vi "Teleop.vi"(10 "Match Info":T1={"Autonomous Elapsed Seconds"=0.0, "TeleOp Elapsed Seconds"=0.0, "Disabled Elapsed Seconds"=0.0, "Visited Autonomous"=FALSE, "Visited TeleOp"=FALSE, "Visited Disabled"=FALSE, "Autonomous Settings"={"Autonomous Style"=enum."Independent", "VI Refnum"=refnum}}, 11 "Call Context":T2) -> ()   [LabVIEW 2014]
doc: "This VI is called for each TeleOp packet received from the DS where the robot is not disabled. It is often used to read from the joysticks and update I/O or to update setpoints for timed control loops. It should complete and return within 20 milliseconds or it may miss DS packets."
uses:
  <vilib>/Rock Robotics/WPI/DriverStation/WPI_DriverStationDerivedRobotMode.ctl
  <vilib>/Rock Robotics/WPI/DriverStation/WPI_DriverStationMatch Info.ctl
  Drivetrain Code/Drivetrain Control.ctl
  Drivetrain Code/Drivetrain Mode.ctl
  Common Code/Change Detect.vi
  Common Code/Change Detect Boolean.vi
  <vilib>/Rock Robotics/WPI/Joystick/WPI_JoystickGetSetRefNum.vi
  Robot Global Data.vi
  <vilib>/Rock Robotics/WPI/Solenoid/Deprecated/WPI_SolenoidSetBool.vi
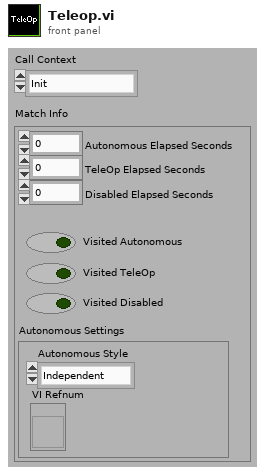
[diagram p1: front panel]
types:
  T1 = typedef "WPI_DriverStationMatch Info.ctl" = cluster{"Autonomous Elapsed Seconds":dbl, "TeleOp Elapsed Seconds":dbl, "Disabled Elapsed Seconds":dbl, "Visited Autonomous":bool, "Visited TeleOp":bool, "Visited Disabled":bool, "Autonomous Settings":cluster{"Autonomous Style":enum16{"Iterative", "Independent"}, "VI Refnum":refnum<vi>}}
  T2 = typedef "WPI_DriverStationDerivedRobotMode.ctl" = enum16{"Init", "Execute", "Stop"}
  T3 = enum16{"0", "1", "2", "3", "4", "5", "6", "7", "8", "9", "A", "B", "C", "D", "E", "F", "G", "H", "I", "J", "K", "L", "M", "N", "O", "P", "Q", "R", "S", "T", "U", "V", "W", "X", "Y", "Z", "F1", "F2", "F3", "F4", "F5", "F6", "F7", "F8", "F9", "F10", "F11", "F12", "F13", "F14", "F15", "ADD", "BACK", "BACKSLASH", "CAPITAL", "COMMA", "DECIMAL", "DELETE", "DIVIDE", "DOWN", "END", "EQUALS", "ESCAPE", "GRAVE (`)", "HOME", "INSERT", "LBRACKET", "LCONTROL", "LEFT", "L ALT", "LSHIFT", "LWIN", "MINUS", "MULTIPLY", "NEXT", "NUMLOCK", "NUMPAD_0", "NUMPAD_1", "NUMPAD_2", "NUMPAD_3", "NUMPAD_4", "NUMPAD_5", "NUMPAD_6", "NUMPAD_7", "NUMPAD_8", "NUMPAD_9", "PAUSE", "PERIOD", "PRIOR (PG UP)", "RBRACKET", "RCONTROL", "RETURN", "RIGHT", "R ALT", "RSHIFT", "RWIN", "SCROLL", "SEMICOLON", "SLASH", "SPACE", "SUBTRACT", "TAB", "UP", "ENTER (num pad)", "' (quote)"}
  T4 = typedef "Drivetrain Mode.ctl" = enum16{"Manual", "Gyro Steer", "Vision Steer", "Drive Distance", "Yaw Rate Compensate"}
  T5 = typedef "Drivetrain Control.ctl" = cluster{"Mode":T4, "Steer":dbl, "Y":dbl, "Heading Target":dbl, "Strafe X":dbl, "Y Target":dbl, "Strafe Target":dbl, "X Max Speed":dbl, "X Min Speed":dbl, "Y Max Speed":dbl, "Y Min Speed":dbl, "Force strafe":bool, "Pivot Speed":dbl}
  T6 = typedef "WPI_JoystickDevRef.ctl" = cluster{"Device":T7}
  T7 = typedef "WPI_JoystickDeviceEnum.ctl" = enum16{"USB 0", "USB 1", "USB 2", "USB 3", "USB 4", "USB 5"}
  T8 = typedef "D-Pad.ctl" = cluster{"Top":bool, "Bottom":bool, "None":bool, "Right":bool, "Left":bool}
  T9 = typedef "Button Cluster.ctl" = cluster{"Buttons[0]":bool, "Buttons[1]":bool, "Buttons[2]":bool, "Buttons[3]":bool, "Buttons[4]":bool, "Buttons[5]":bool, "Buttons[6]":bool, "Buttons[7]":bool, "Buttons[8]":bool, "Buttons[9]":bool}
  T10 = typedef "Axes Cluster.ctl" = cluster{"Axes[0]":dbl, "Axes[1]":dbl, "Axes[2]":dbl, "Axes[3]":dbl, "Axes[4]":dbl, "Axes[5]":dbl, "Axes[6]":dbl, "Axes[7]":dbl, "Axes[8]":dbl}
  T11 = typedef "Dashboard Control Data.ctl" = cluster{"Cam Exposure":dbl, "Go to angle":dbl, "Steer PID Gains":cluster{"proportional gain (Kc)":dbl, "integral time (Ti, min)":dbl, "derivative time (Td, min)":dbl}, "Steer PID output Range":cluster{"output high":dbl, "output low":dbl}, "Pressure m \nValue":dbl, "Pressure b \nValue":dbl, "Roller Command Cluster ":T12, "Elevator":T13, "Encoder Control":T15, "Auton Settings":cluster{"Drive Dist Window Size":dbl}, "Drivetrain Settings":T16, "Lance":T17}
  T12 = typedef "Roller Control.ctl" = cluster{"Intake Speed":dbl, "Turn In Speed":dbl, "Unload Speed":dbl, "Turn Out Speed":dbl, "Ping Align Tolerance":dbl, "Tote Range Threshold":dbl, "Right Pot 0":dbl, "Pot Threshold":dbl, "Left Pot 0":dbl, "Right Pot Scale":dbl, "Left Pot Scale":dbl, "Min Elevator Height":dbl, "Eject Time":dbl, "Eject US Threshold":dbl, "Anti-Twitch Time":u32, "Ping Caring Threshold":dbl, "Pot Diff Threshold":dbl, "Pinch Sustain":u32, "Absorb Give Up Threshold":dbl, "Untip In Threshold":dbl, "Untip Grab Range":dbl, "Ultrasonic Hold Time":u32, "Landscape Absorb Time":u32, "Pot Use Wait Time":u32, "Can Turn Stop Range":dbl, "HP Load Speed":dbl, "Stick Multiplier":dbl, "Coop Eject Speed":dbl}
  T13 = typedef "Elevator DB Control.ctl" = cluster{"PID Output Range":cluster{"output high":dbl, "output low":dbl}, "PID gains":cluster{"proportional gain (Kc)":dbl, "integral time (Ti, min)":dbl, "derivative time (Td, min)":dbl}, "Height Tolerance":sgl, " Encoder Constant":dbl, "Eject Time":sgl, "Zeroing Speed":sgl, "Presets":T14, "Ping Detect Threshold":sgl, "Trashcan Detect Threshold":sgl, "Zero Filter Time":dbl, "Stabilizer Open Time":dbl, "Zero Creep Speed":dbl, "Max Current":dbl, "Current Trip Time":dbl, "Abort Pitch":dbl, "Finger m":dbl, "Finger b":dbl, "Finger max ":dbl, "Finger Stabilizer":dbl, "Finger Store":dbl, "Finger Stop Store":dbl, "Stabilizer Close Time":dbl, "Finger min":dbl, "Unstick gain":dbl, "Full Detect Max":dbl}
  T14 = typedef "Elevator Presets.ctl" = cluster{"Pickup 2 w/ Tote":sgl, "Pickup 2 w/ Trashcan":sgl, "Pickup 3 w/ Tote":sgl, "Pickup 3 w/ Trashcan":sgl, "Bottom":sgl, "Pickup 1 w/ Tote":sgl, "Pickup Trashcan":sgl, "Pickup 1 w/ Trashcan":sgl, "Eject":sgl, "Hold Low":sgl, "Step add height":sgl, "Untip Lift":dbl, "Drop Stack":dbl, "HP Load Hold":dbl, "HP Load Drop":dbl, "HP Load Hold Can":dbl, "Store can max":dbl, "HP Drag Score":dbl, "HP Drag Finish":dbl, "Finger trashcan avoid":dbl, "Full":dbl}
  T15 = typedef "Encoder Control.ctl" = cluster{"Left Tick Constant":dbl, "Right Tick Constant":dbl, "Center Tick Constant":dbl, "Reset?":bool, "Y Dist":cluster{"PID gains":cluster{"proportional gain (Kc)":dbl, "integral time (Ti, min)":dbl, "derivative time (Td, min)":dbl}}, "X Dist":cluster{"PID gains":cluster{"proportional gain (Kc)":dbl, "integral time (Ti, min)":dbl, "derivative time (Td, min)":dbl}}, "Y Stop Thresh":dbl, "Y Stop Speed":dbl, "X Stop Thresh":dbl, "X Stop Speed":dbl}
  T16 = typedef "Drivetrain Settings.ctl" = cluster{"Gyro Tolerance":sgl, "Strafe Correct max steer":sgl, "Strafe Timer Wait":sgl, "Throttle Ramp (ms)":sgl, "Strafe Ramp (ms)":sgl, "Angular rate compensation":bool, "Throttle to Rate Scale":sgl, "Rate compensation gain":sgl, "Creep Steer":sgl, "Creep Throttle":sgl}
  T17 = typedef "Pike DB Controls.ctl" = cluster{"Down Speed":dbl, "Up Speed":dbl, "Max Down Time":dbl, "Max Up Time":dbl, "Current Limit":dbl}
  T18 = typedef "WPI_SolenoidDevRef.ctl" = cluster{"DevStatus":errorcluster, "Pneumatics Control Module":u8, "Forward Solenoid Channel":T19, "Reverse Solenoid Channel":T19}
  T19 = typedef "WPI_SolenoidChannel.ctl" = enum8{"Solenoid 0", "Solenoid 1", "Solenoid 2", "Solenoid 3", "Solenoid 4", "Solenoid 5", "Solenoid 6", "Solenoid 7", "Invalid"}
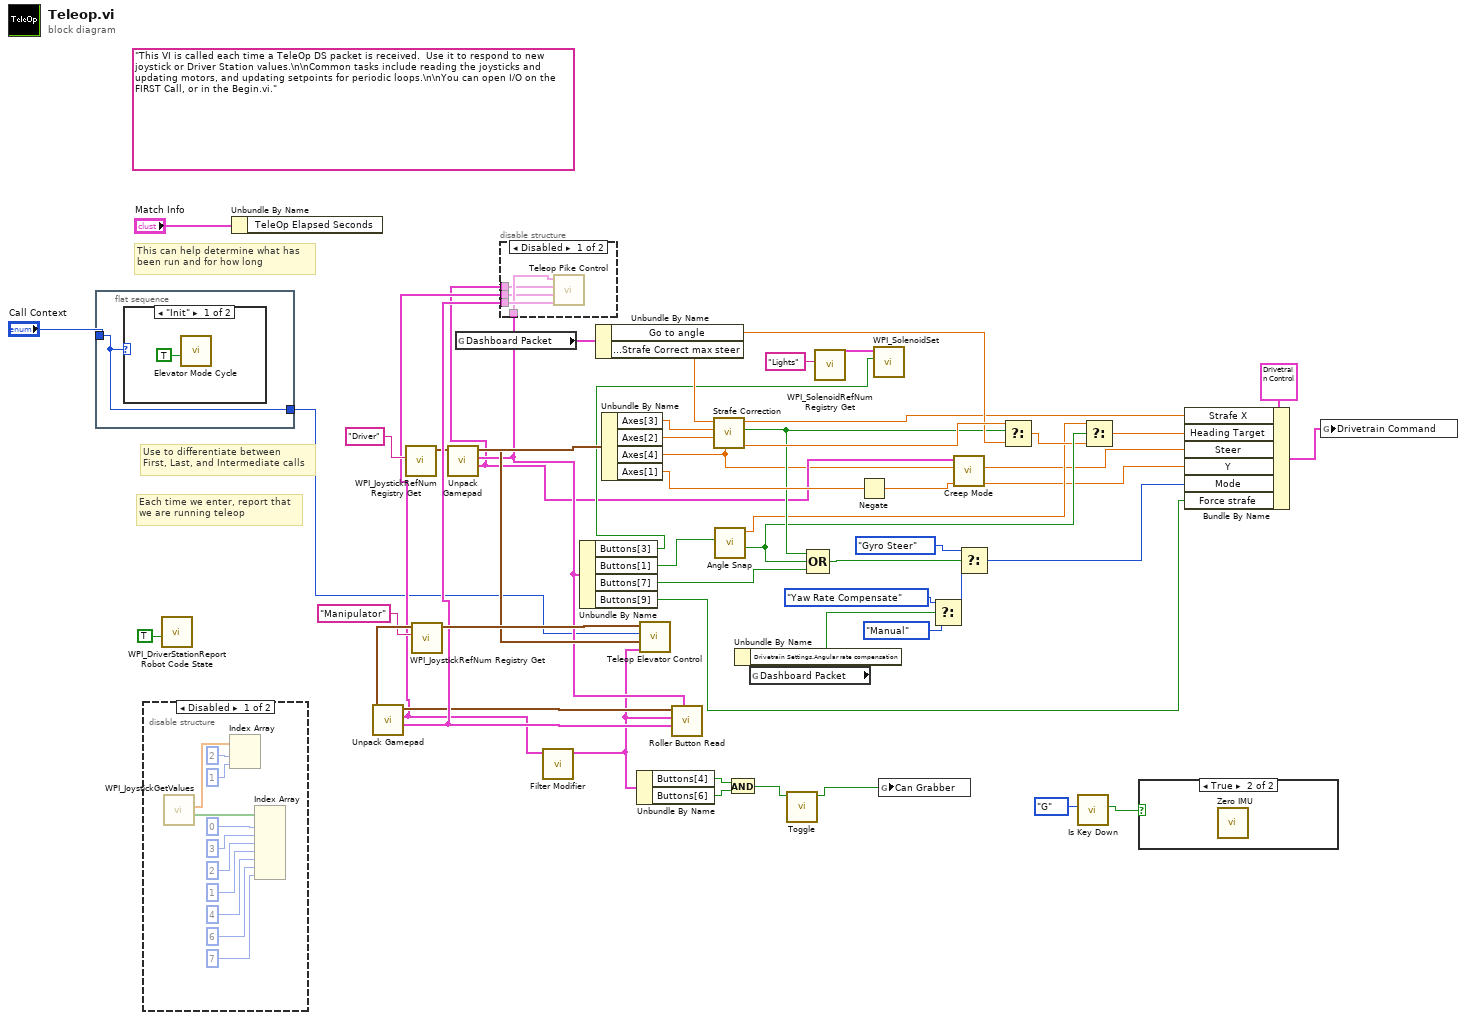
[diagram p0: block diagram]
diagram:
  (unwired) "This VI is called each time a TeleOp DS packet is received.  Use it to respond to new joystick or Driver Station values.\n\nCommon tasks include reading the joysticks and updating motors, and updating setpoints for periodic loops.\n\nYou can open I/O on the FIRST Call, or in the Begin.vi."
  # "Each time we enter, report that\nwe are running teleop"
  # "Use to differentiate between\nFirst, Last, and Intermediate calls"
  # "This can help determine what has\nbeen run and for how long"
  n1 = flat-sequence {
    tunnel: "Call Context" -> [w55]
    tunnel: [w55] -> w1
    frame #0 {
      n2 = case shown="\"Init\"" w55 {
        frame "Init" {
          n3 = call "Elevator Mode Cycle.vi"("Set to Auto"=TRUE) -> ()  [unwired: 10 in, 1 out]
        }
        frame Default {
        }
      }
    }
  }
  n4 = disable-structure shown="Disabled" {
    frame Disabled {
      n5 = call <vilib>:"WPI_JoystickGetValues.vi"() -> ("Buttons"=w64:bool[], "Axes"=w67:dbl[])  [unwired: 7 in, 3 out]
      n6 = Index Array(array=w67, index #1=2 ("index"), index #2=1 ("index")) -> ()  [unwired: 2 out]
      n7 = Index Array(array=w64, index #1=0 ("index"), index #2=3 ("index"), index #3=2 ("index"), index #4=1 ("index"), index #5=4 ("index"), index #6=6 ("index"), index #7=7 ("index")) -> ()  [unwired: 7 out]
    }
    frame Enabled {
    }
  }
  n8 = call <vilib>:"WPI_DriverStationReport Robot Code State.vi"("TeleOp"=TRUE ("Autonomous")) -> ()  [unwired: 10 in, 1 out]
  n9 = Unbundle By Name("Match Info") -> ()  [unwired: 1 out]
  n10 = call <vilib>:"WPI_JoystickRefNum Registry Get.vi"("refnum name"="Driver") -> ("JoystickDevRef"=w37:T6)  [unwired: 9 in, 1 out]
  n11 = call <vilib>:"WPI_JoystickRefNum Registry Get.vi"("refnum name"="Manipulator") -> ("JoystickDevRef"=w50:T6)  [unwired: 9 in, 1 out]
  n12 = call "Unpack Gamepad.vi"("JoystickDevRef"=w50) -> ("D-Pad"=w49:T8, "Button Cluster"=w34:T9, "Axes"=w48:T10)  [unwired: 8 in]
  n13 = call "Unpack Gamepad.vi"("JoystickDevRef"=w37) -> ("D-Pad"=w7:T8, "Button Cluster"=w36:T9, "Axes"=w42:T10)  [unwired: 8 in]
  n14 = global read "Robot Global Data.vi" "Dashboard Packet"() -> (w31:T11)
  n15 = disable-structure shown="Disabled" {
    disable-tunnel: w49 -> [w71 _]
    disable-tunnel: w36 -> [w70 _]
    disable-tunnel: w34 -> [w69 _]
    disable-tunnel: w7 -> [w68 _]
    frame Disabled {
      n16 = call "Teleop Pike Control.vi"("Manipulator D-Pad"=w71, "Manipulator Buttons"=w69, "Driver D-Pad"=w68, "Driver Buttons"=w70) -> ()  [unwired: 8 in]
    }
    frame Enabled {
    }
  }
  n17 = call "Filter Modifier.vi"("Button Cluster 1"=w34) -> ("Button Cluster Out"=w35:T9)  [unwired: 10 in]
  n18 = Unbundle By Name(w36) -> ("Buttons[3]"=w9:bool, "Buttons[1]"=w19:bool, "Buttons[7]"=w39:bool, "Buttons[9]"=w8:bool)
  n19 = Unbundle By Name(w31) -> ("Go to angle"=w33:dbl, "Drivetrain Settings.Strafe Correct max steer"=w32:sgl)
  n20 = Unbundle By Name(w42) -> ("Axes[3]"=w45:dbl, "Axes[2]"=w44:dbl, "Axes[4]"=w4:dbl, "Axes[1]"=w43:dbl)
  n21 = Unbundle By Name(w35) -> ("Buttons[4]"=w30:bool, "Buttons[6]"=w29:bool)
  n22 = call "Teleop Elevator Control.vi"("Button Cluster"=w35, "Driver Joystick"=w37, "Call Context"=w1, "Manipulator Joystick"=w50) -> ()  [unwired: 8 in]
  n23 = call "Roller Button Read.vi"("Driver Button Cluster"=w36, "D-Pad"=w49, "Button Cluster"=w35, "Axes"=w48) -> ()  [unwired: 8 in]
  n24 = call "Strafe Correction.vi"("Steer"=w4, "L Trigger"=w44, "R Trigger"=w45, "Max Steer"=w32) -> ("Angle"=w40:dbl, "Gyro Steer"=w18:bool, "Strafe Out"=w22:dbl)  [unwired: 5 in]
  n25 = call "Angle Snap.vi"("Enable?"=w19) -> ("Gyro Steer?"=w17:bool, "Heading Out"=w15:dbl)  [unwired: 9 in]
  n26 = And(x=w30, y=w29) -> (x .and. y?=w28:bool)
  n27 = global read "Robot Global Data.vi" "Dashboard Packet"() -> (w21:T11)
  n28 = Unbundle By Name(w21) -> ("Drivetrain Settings.Angular rate compensation"=w20:bool)
  n29 = call "Toggle.vi"("In"=w28) -> ("Toggled"=w27:bool)  [unwired: 10 in]
  n30 = Compound Arithmetic op=OR(w18, w17, w39) -> (w38:bool)
  n31 = call <vilib>:"WPI_SolenoidRefNum Registry Get.vi"("refnum name"="Lights") -> ("SolenoidDevRef"=w11:T18)  [unwired: 9 in, 1 out]
  n32 = Negate(x=w43) -> (-x=w5:dbl)
  n33 = call-poly <vilib>:"WPI_SolenoidSet.vi"("Value"=w9, "SolenoidDevRef"=w11) -> ()  [unwired: 8 in, 2 out]
  n34 = global write "Robot Global Data.vi" "Can Grabber"(w27) -> ()
  n35 = Select(t=Drivetrain_Mode."Yaw Rate Compensate" ("Mode"), s=w20, f=Drivetrain_Mode."Manual" ("Mode")) -> (s? t:f=w24:T4)
  n36 = call "Creep Mode.vi"("Throttle In"=w5, "Steer In"=w4, "D-Pad"=w7) -> ("Throttle Out"=w6:dbl, "Steer Out"=w3:dbl)  [unwired: 7 in]
  n37 = Select(t=Drivetrain_Mode."Gyro Steer" ("Mode"), s=w38, f=w24) -> (s? t:f=w23:T4)
  n38 = Select(t=w40, s=w18, f=w33) -> (s? t:f=w16:dbl)
  n39 = call "Is Key Down.vi"("Key"=T3."G") -> ("Key Down?"=w13:bool)  [unwired: 10 in]
  n40 = Select(t=w15, s=w17, f=w16) -> (s? t:f=w14:dbl)
  n41 = case shown="True" w13 {
    frame False {
    }
    frame True {
      n42 = call "Zero IMU.vi"() -> ()  [unwired: 12 in]
    }
  }
  n43 = Bundle By Name(cluster=T5 {"Mode"=enum."Gyro Steer", "Steer"=0.0, "Y"=0.0, "Heading Target"=0.0, "Strafe X"=0.0, "Y Target"=0.0, "Strafe Target"=0.0, "X Max Speed"=0.0, "X Min Speed"=0.0, "Y Max Speed"=0.0, "Y Min Speed"=0.0, "Force strafe"=FALSE, "Pivot Speed"=0.0} ("Drivetrain Command"), "Strafe X"=w22, "Heading Target"=w14, "Steer"=w3, "Y"=w6, "Mode"=w23, "Force strafe"=w8) -> (w52:T5)
  n44 = global write "Robot Global Data.vi" "Drivetrain Command"(w52) -> ()
